vi "estrcutura de casos.vi"() -> ()   [LabVIEW 2020]
panel:
  in  "Boolean 2":bool
  out "x+y":dbl
  in  "y":dbl
  in  "x":dbl
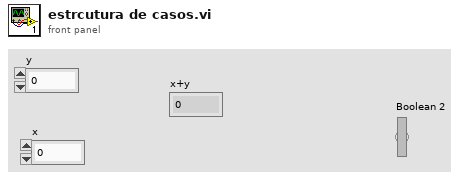
[diagram p1: front panel]
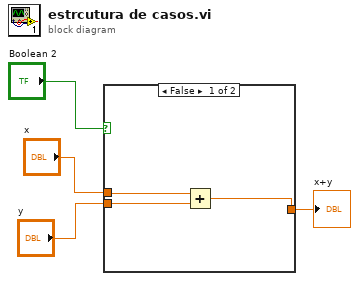
[diagram p0: block diagram]
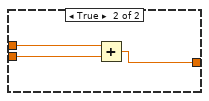
[diagram p2: hidden frame]
diagram:
  n1 = case shown="False" "Boolean 2" {
    tunnel: "x" -> [w7 w10]
    tunnel: "y" -> [w6 w9]
    tunnel: [w5 w8] -> w2
    frame False {
      n2 = Add(x=w7, y=w6) -> (x+y=w5:dbl)
    }
    frame True {
      n3 = Add(x=w10, y=w9) -> (x+y=w8:dbl)
    }
  }
  "x+y" <- w2
